vi "mkGetSetInFrameCounter.vi"(9 "Set? (F)":bool, 10 "Enable in-frame counter (T)":bool=TRUE, 11 "IMAQ Refnum in":refnum<k11>) -> (2 "Enable in-frame counter (out)":bool, 3 "IMAQ Refnum out":refnum<k11>)   [LabVIEW 2011]
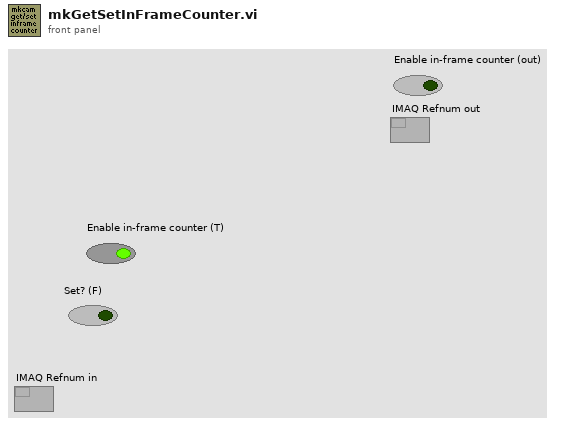
[diagram p1: front panel]
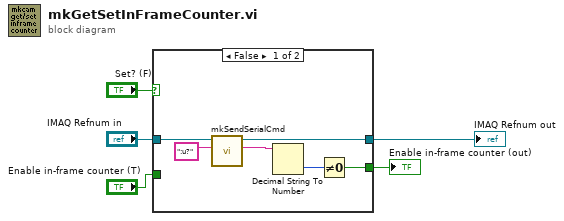
[diagram p0: block diagram]
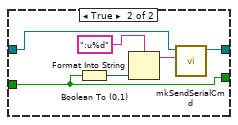
[diagram p2: hidden frame]
diagram:
  n1 = case shown="False" "Set? (F)" {
    tunnel: "Enable in-frame counter (T)" -> [_ w12]
    tunnel: "IMAQ Refnum in" -> [w9 w14]
    tunnel: [w11 w13] -> w1
    tunnel: [w6 w12] -> w2
    frame False {
      n2 = call "mkSendSerialCmd.vi"("String"=":u?", "IMAQ Refnum in"=w9) -> ("String Read"=w8:string, "IMAQ Refnum out"=w11:refnum<k11>)  [unwired: 6 in, 2 out]
      n3 = Decimal String To Number(string=w8) -> (number=w7:i32)  [unwired: 2 in, 1 out]
      n4 = Not Equal To 0?(x=w7) -> (x != 0?=w6:bool)
    }
    frame True {
      n5 = Boolean To (0,1)(Boolean=w12) -> (0, 1=w16:i16)
      n6 = Format Into String(format string=":u%d", w16) -> (resulting string=w15:string)  [unwired: 2 in, 1 out]
      n7 = call "mkSendSerialCmd.vi"("String"=w15, "IMAQ Refnum in"=w14) -> ("IMAQ Refnum out"=w13:refnum<k11>)  [unwired: 6 in, 3 out]
    }
  }
  "Enable in-frame counter (out)" <- w2
  "IMAQ Refnum out" <- w1
